vi "Create Pump Command.vi"(8 "error in (no error)":errorcluster, 11 "Section Ptr":T6 format="%.0x") -> (0 "error out":errorcluster, 2 "Command Pump":T1={"Mode"=enum."Off", "Digital Input"=enum."Unused", "Default Profile Index"=0, "Cal Freq [Hz]"=0.0, "Cal Duration [s]"=0.0, "Cal Increment [s]"=0.0, "Cal Pulses"=0, "TMP Command Sequence"=[{"Duration [s]"=0.0, "Level"=FALSE, "Run/Stop"=FALSE, "Profile Index"=0}, {"Duration [s]"=0.0, "Level"=FALSE, "Run/Stop"=FALSE, "Profile Index"=0}, {"Duration [s]"=0.0, "Level"=FALSE, "Run/Stop"=FALSE, "Profile Index"=0}, {"Duration [s]"=0.0, "Level"=FALSE, "Run/Stop"=FALSE, "Profile Index"=0}, {"Duration [s]"=0.0, "Level"=FALSE, "Run/Stop"=FALSE, "Profile Index"=0}, {"Duration [s]"=0.0, "Level"=FALSE, "Run/Stop"=FALSE, "Profile Index"=0}, {"Duration [s]"=0.0, "Level"=FALSE, "Run/Stop"=FALSE, "Profile Index"=0}, {"Duration [s]"=0.0, "Level"=FALSE, "Run/Stop"=FALSE, "Profile Index"=0}, {"Duration [s]"=0.0, "Level"=FALSE, "Run/Stop"=FALSE, "Profile Index"=0}, {"Duration [s]"=0.0, "Level"=FALSE, "Run/Stop"=FALSE, "Profile Index"=0}, {"Duration [s]"=0.0, "Level"=FALSE, "Run/Stop"=FALSE, "Profile Index"=0}, {"Duration [s]"=0.0, "Level"=FALSE, "Run/Stop"=FALSE, "Profile Index"=0}, {"Duration [s]"=0.0, "Level"=FALSE, "Run/Stop"=FALSE, "Profile Index"=0}, {"Duration [s]"=0.0, "Level"=FALSE, "Run/Stop"=FALSE, "Profile Index"=0}, {"Duration [s]"=0.0, "Level"=FALSE, "Run/Stop"=FALSE, "Profile Index"=0}, {"Duration [s]"=0.0, "Level"=FALSE, "Run/Stop"=FALSE, "Profile Index"=0}], "EPT TDC Offset [CAD]"=0.0, "EPT Window Start [DBTDC]"=0.0, "EPT Window End [DBTDC]"=0.0, "EPT Angles"=[{"Enable"=FALSE, "Timing [DBTDC]"=0.0, "Duration [s]"=0.0, "Profile Index"=0}, {"Enable"=FALSE, "Timing [DBTDC]"=0.0, "Duration [s]"=0.0, "Profile Index"=0}, {"Enable"=FALSE, "Timing [DBTDC]"=0.0, "Duration [s]"=0.0, "Profile Index"=0}, {"Enable"=FALSE, "Timing [DBTDC]"=0.0, "Duration [s]"=0.0, "Profile Index"=0}, {"Enable"=FALSE, "Timing [DBTDC]"=0.0, "Duration [s]"=0.0, "Profile Index"=0}, {"Enable"=FALSE, "Timing [DBTDC]"=0.0, "Duration [s]"=0.0, "Profile Index"=0}, {"Enable"=FALSE, "Timing [DBTDC]"=0.0, "Duration [s]"=0.0, "Profile Index"=0}, {"Enable"=FALSE, "Timing [DBTDC]"=0.0, "Duration [s]"=0.0, "Profile Index"=0}], "EPT Skip Fire"=FALSE, "EPT Skip Index"=0, "EPT Precharge Duration [s]"=0.0, "EPT Precharge Profile Index"=0} {"EPT Precharge Profile Index" max=15; "EPT Precharge Duration [s]" min=0 format="%#_4p"; "Default Profile Index" max=15; "Cal Increment [s]" format="%#_3p"; "TMP Command Sequence"."Profile Index" max=7; "TMP Command Sequence"."Duration [s]" min=0 max=100 format="%#_3p"; "Cal Pulses" max=511; "EPT Skip Index" max=7; "EPT Angles"."Profile Index" max=7; "EPT Angles"."Duration [s]" min=0 max=100 format="%#_3p"; "Cal Duration [s]" format="%#_3p"; "Cal Freq [Hz]" format="%#_3p"}, 3 "Parent Ref out":T6 format="%.0x")   [LabVIEW 2016, in "DCM System Explorer.lvlib"]
uses:
  DCM System Explorer.lvlib
  <vilib>/NI Veristand/Custom Device API/Custom Device Item Ref.ctl
  <vilib>/Powertrain Controls/Device Drivers/DCM/DI/RT/Command.ctl
  <vilib>/Powertrain Controls/Device Drivers/DCM/DI/FPGA/Mode.ctl
  <vilib>/Powertrain Controls/Device Drivers/DCM/Rev0/FPGA/Digital Channel.ctl
  <vilib>/Powertrain Controls/Device Drivers/DCM/DI/RT/Command Sequence.ctl
  <vilib>/Powertrain Controls/Device Drivers/DCM/DI/RT/Angle Control.ctl
  <vilib>/NI Veristand/Custom Device API/Custom Device Channel Type.ctl
  <vilib>/NI VeriStand/Custom Device API/Custom Device API.lvlib
  <vilib>/Powertrain Controls/Device Drivers/DCM/DI/RT/DCM - RT - DI.lvlib
  <vilib>/Powertrain Controls/Device Drivers/DCM/DI/FPGA/DCM - FPGA - DI.lvlib
  <vilib>/Powertrain Controls/Device Drivers/DCM/Rev0/FPGA/DCM - FPGA.lvlib
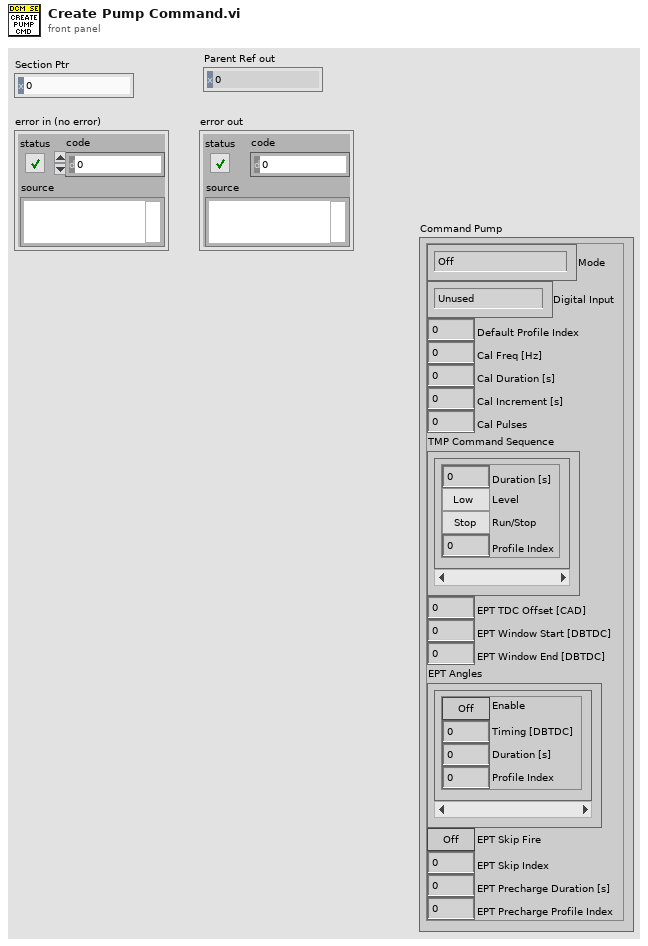
[diagram p1: front panel]
types:
  T1 = typedef "DCM - RT - DI.lvlib/Command.ctl" = cluster{"Mode":T2, "Digital Input":T3, "Default Profile Index":u8, "Cal Freq [Hz]":sgl, "Cal Duration [s]":sgl, "Cal Increment [s]":sgl, "Cal Pulses":u16, "TMP Command Sequence":T4[], "EPT TDC Offset [CAD]":sgl, "EPT Window Start [DBTDC]":sgl, "EPT Window End [DBTDC]":sgl, "EPT Angles":T5[], "EPT Skip Fire":bool, "EPT Skip Index":u8, "EPT Precharge Duration [s]":sgl, "EPT Precharge Profile Index":u8}
  T2 = typedef "DCM - FPGA - DI.lvlib/Mode.ctl" = enum8{"Off", "Direct", "Calibration", "Triggered Multi-Pulse", "Engine Position Tracking"}
  T3 = typedef "DCM - FPGA.lvlib/Digital Channel.ctl" = enum8{"Unused", "User OS", "Diff IO 1", "Diff IO 2", "Diff IO 3", "Diff IO 4", "Diff IO 5", "Diff IO 6", "Diff IO 7", "Diff IO 8", "Aux 1", "Aux 2", "Aux 3", "Aux 4", "Aux 5", "Aux 6", "Aux 7", "Aux 8", "Aux 9", "Aux 10", "Aux 11", "Aux 12", "Aux 13", "Aux 14", "Aux 15", "Aux 16"}
  T4 = typedef "DCM - RT - DI.lvlib/Command Sequence.ctl" = cluster{"Duration [s]":sgl, "Level":bool, "Run/Stop":bool, "Profile Index":u8}
  T5 = typedef "DCM - RT - DI.lvlib/Angle Control.ctl" = cluster{"Enable":bool, "Timing [DBTDC]":sgl, "Duration [s]":sgl, "Profile Index":u8}
  T6 = typedef "Custom Device API.lvlib/Custom Device Item Ref.ctl" = u64
  T7 = typedef "Custom Device API.lvlib/Custom Device Channel Type.ctl" = enum16{"Input", "Output"}
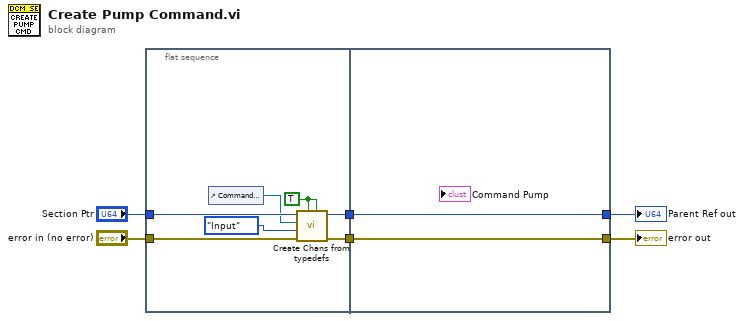
[diagram p0: block diagram]
diagram:
  n1 = flat-sequence {
    tunnel: [w9] -> w2
    tunnel: "Section Ptr" -> [w11]
    tunnel: "error in (no error)" -> [w10]
    tunnel: [w8] -> w1
    tunnel: [w15] -> w4
    tunnel: [w14] -> w3
    tunnel: w2 -> [w15]
    tunnel: w1 -> [w14]
    frame #0 {
      w12 = TRUE ("Prevent overwrite? (F)")
      n2 = control-ref of="Command Pump"() -> (w7:refnum<vi>)
      n3 = call "Create Chans from typedefs.vi"("Default from text? (F)"=w12, "Prevent overwrite? (F)"=w12, "error in"=w10, "Type"=Custom_Device_Channel_Type."Input", "Ctl Ref"=w7, "Section Ref in"=w11) -> ("error out"=w8:errorcluster, "Section Ref out"=w9:T6)  [unwired: 3 in, 1 out]
    }
    frame #1 {
    }
  }
  "Parent Ref out" <- w4
  "error out" <- w3
